vi "Create Channel Task.vi"(8 "error in":errorcluster, 10 "SQL query":string="SELECT max(MaximumVoltage),max(MinimumVoltage), max(TerminalConfiguration),max(SampleRate) FROM ltt.daq_configuration \nWhere ChannelType='Waveform_Output' and Enabled=1;", 11 "NI Waveform Output in":refnum<class "NI Waveform Output.lvclass">) -> (0 "error out":errorcluster, 3 "NI Waveform Output out":refnum<class "NI Waveform Output.lvclass">)   [LabVIEW 2023, in "HardwareAbstractionLayer_LVOOP.lvlib" / "NI Waveform Output.lvclass"]
doc: "This VI Analog Output Physical Channel Based DAQmx Create Channel"
uses:
  NI Waveform Output.lvclass
  NI Waveform Output.lvclass/NI Waveform Output.ctl
  <vilib>/DAQmx/create/channels.llb/DAQmx Create Channel (AO-Voltage-Basic).vi
  <vilib>/DAQmx/configure/timing.llb/DAQmx Timing (Sample Clock).vi
  Database/Database.lvclass
panel:
  # "SELECT max(MaximumVoltage),max(MinimumVoltage), max(TerminalConfiguration),max(SampleRate) FROM ltt.daq_configuration \nWhere ChannelType='Waveform_Output' and Enabled=1;"
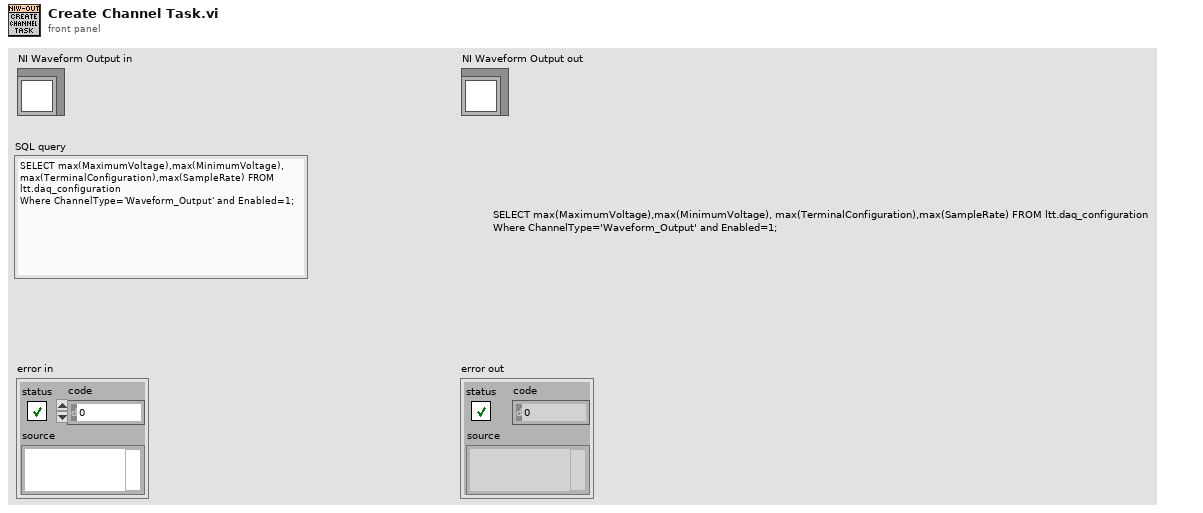
[diagram p1: front panel]
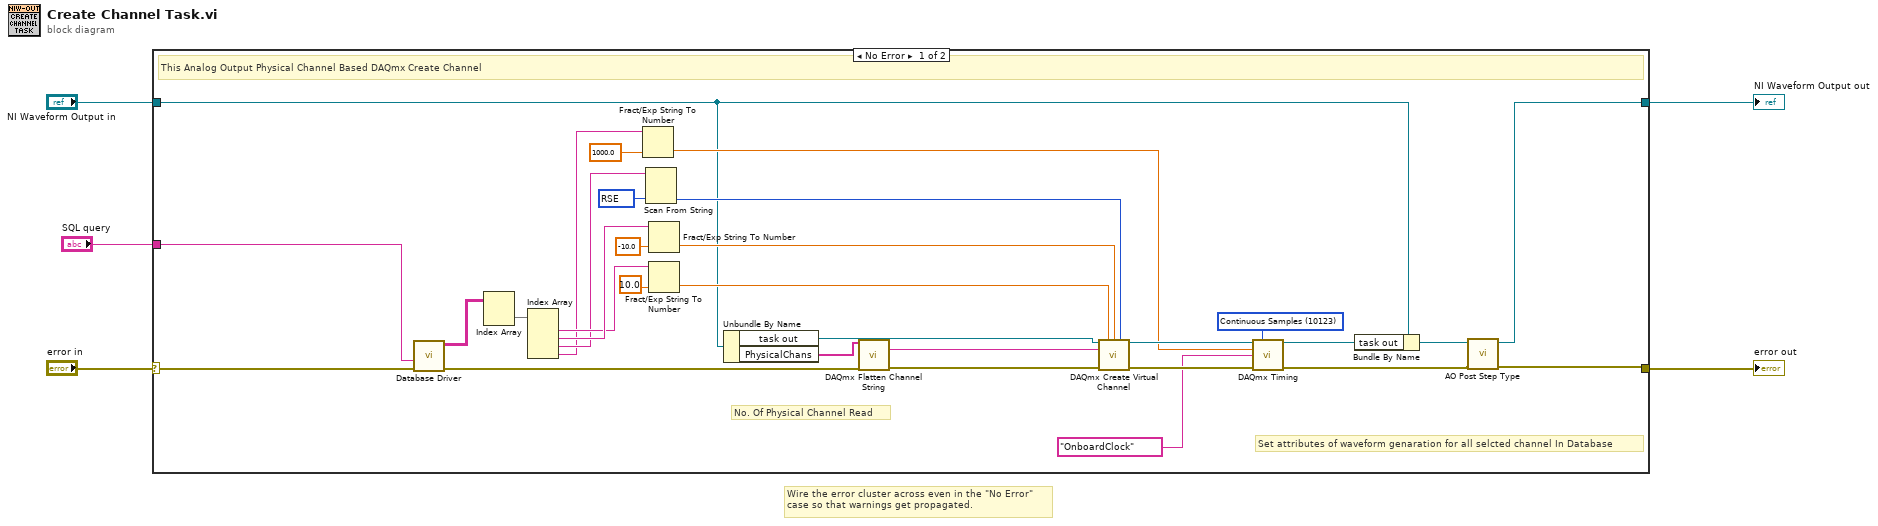
[diagram p0: block diagram]
diagram:
  # "Wire the error cluster across even in the \"No Error\"\ncase so that warnings get propagated."
  n1 = case shown="No Error" "error in" {
    selector: "error in" -> [w15 w38]
    tunnel: [w7 w38] -> w4
    tunnel: [w9 w37] -> w2
    tunnel: "NI Waveform Output in" -> [w11 w37]
    tunnel: "SQL query" -> [w6 _]
    frame No Error {
      w17 = 10123 items=["Finite Samples"=10178, "Continuous Samples"=10123, "Hardware Timed Single Point"=12522] ("sample mode")
      w33 = 10083 items=["Default"=-1, "RSE"=10083, "NRSE"=10078, "Differential"=10106, "Pseudodifferential"=12529] ("input terminal configuration")
      # "Set attributes of waveform genaration for all selcted channel In Database"
      # "No. Of Physical Channel Read"
      # "This Analog Output Physical Channel Based DAQmx Create Channel"
      n2 = call "Database Driver.vi"("error in"=w15, "SQL query"=w6) -> ("error out"=w13:errorcluster, "data"=w14:string[][])  [unwired: 6 in, 2 out]
      n3 = Index Array(array=w14) -> (element=w34:string[])  [unwired: 2 in]
      n4 = Index Array(array=w34) -> (element #1=w35:string, element #2=w36:string, element #3=w27:string, element #4=w19:string)  [unwired: 4 in]
      n5 = Fract/Exp String To Number(string=w19, default (0 dbl)=1000.0 ("rate")) -> (number=w18:dbl)  [unwired: 2 in, 1 out]
      n6 = Scan From String(input string=w27, default 1=w33) -> (output 1=w28:i32)  [unwired: 3 in, 3 out]
      n7 = Fract/Exp String To Number(string=w36, default (0 dbl)=-10.0 ("maximum value")) -> (number=w29:dbl)  [unwired: 2 in, 1 out]
      n8 = Fract/Exp String To Number(string=w35, default (0 dbl)=10.0 ("maximum value")) -> (number=w30:dbl)  [unwired: 2 in, 1 out]
      n9 = Unbundle By Name(w11) -> ("task out"=w23:refnum<k21>, "PhysicalChans"=w25:tag[])
      n10 = call <vilib>:"DAQmx Flatten Channel String.vi"("names in"=w25, "error in"=w13) -> ("names out"=w24:string, "error out"=w26:errorcluster)  [unwired: 12 in]
      n11 = call-poly <vilib>:"DAQmx Create Virtual Channel.vi"("task in"=w23, "maximum value"=w30, "minimum value"=w29, "output terminal configuration"=w28, "physical channels"=w24, "error in"=w26) -> ("task out"=w21:refnum<k21>, "error out"=w22:errorcluster)  [unwired: 8 in]
      n12 = call-poly <vilib>:"DAQmx Timing.vi"("task/channels in"=w21, "sample mode"=w17, "rate"=w18, "source"=tag "OnboardClock", "error in"=w22) -> ("task out"=w16:refnum<k21>, "error out"=w8:errorcluster)  [unwired: 9 in]
      n13 = Bundle By Name(cluster=w11, "task out"=w16) -> (w10:refnum<class "NI Waveform Output.lvclass">)
      n14 = call-dynamic "AO Post Step Type.vi"("error in (no error)"=w8, "NI Waveform Output in"=w10) -> ("error out"=w7:errorcluster, "NI Waveform Output out"=w9:refnum<class "NI Waveform Output.lvclass">)  [unwired: 7 in, 1 out]
    }
    frame Error {
    }
  }
  "error out" <- w4
  "NI Waveform Output out" <- w2
